vi "File Read.vi"(8 "Default Value":dbl, 9 "key":string, 10 "section":string, 11 "Mode":enum16{"Init", "Run", "End"}(ring)) -> (2 "Output Value":dbl format="%.2f")   [LabVIEW 2013]
uses:
  <vilib>/Utility/config.llb/Read Key (Double).vi
  <vilib>/Utility/config.llb/NI_LVConfig.lvlib
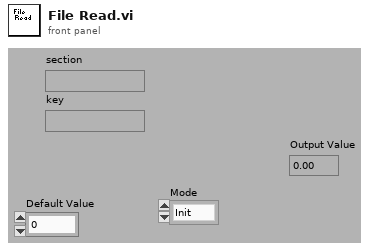
[diagram p1: front panel]
types:
  T1 = typedef "NI_LVConfig.lvlib/Config Data RefNum.ctl" = refnum<k1>
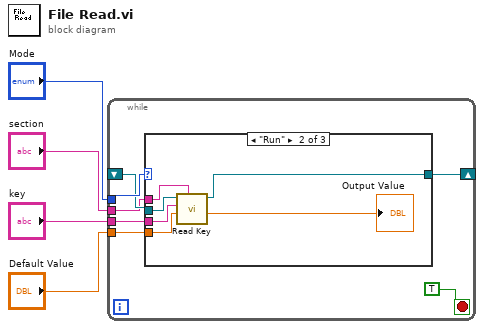
[diagram p0: block diagram]
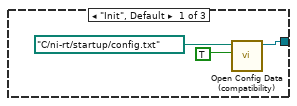
[diagram p2: hidden frame]
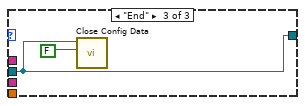
[diagram p3: hidden frame]
diagram:
  n1 = while {
    tunnel: "Mode" -> [w10]
    shift-right: [w9] -> _
    shift-left: _ -> [w8]
    tunnel: "section" -> [w7]
    tunnel: "key" -> [w6]
    tunnel: "Default Value" -> [w5]
    stop <- TRUE stop-if-true
    n2 = case shown="\"Run\"" w10 {
      tunnel: [w13 w19 w22] -> w9
      tunnel: w8 -> [_ w20 w22]
      tunnel: w7 -> [_ w18 _]
      tunnel: w6 -> [_ w17 _]
      tunnel: w5 -> [_ w16 _]
      frame "Init", Default {
        n3 = call <vilib>:"Open Config Data (compatibility).vi"("create file if necessary (T)"=TRUE ("create file if necessary? (T)"), "configuration file path"=path "C:/ni-rt/startup/config.txt") -> ("refnum"=w13:T1)  [unwired: 7 in, 2 out]
      }
      frame "Run" {
        n4 = call-poly <vilib>:"Read Key.vi"("section"=w18, "default value"=w16, "key"=w17, "refnum"=w20) -> ("value"=→"Output Value":dbl, "refnum out"=w19:T1)  [unwired: 1 in, 5 out]
      }
      frame "End" {
        n5 = call <vilib>:"Close Config Data.vi"("write file if changed (T)"=FALSE ("write configuration file? (T)"), "refnum"=w22) -> ()  [unwired: 1 in, 9 out]
      }
    }
  }
